vi "getOutputGain.vi"(8 "error in (no error)":errorcluster, 11 "Instrument.LockinAPI in":refnum<class "Instrument.LockinAPI.lvclass">) -> (0 "error out":errorcluster, 2 "OutputGain":dbl[](array[numeric]), 3 "Instrument.LockinAPI out":refnum<class "Instrument.LockinAPI.lvclass">)   [LabVIEW 2019, in "Instrument.LockinAPI.lvclass"]
doc: "API to get the AI waveforms.\n\nIf address=\"\", this API reads from localhost\nIf address is remote lockin, you need to add this computer to allowed whitelist on the lockin computer you are trying to access."
uses:
  Instrument.LockinAPI.lvclass
  C:/Users/patrick/Documents/GitHub/Instrument-Framework/lvsrc/Framework/Instrument/Instrument.lvclass
  Typedefs/LockinAPI.Commands--Enum.ctl
  00037c6a-def5-4a33-8a82-3535220e14b4.vi
  00037c6a-def5-4a33-8a82-3535220e14b4.vi/72857e9d-b6a5-4918-84de-0a0220085fa5.vi
  00037c6a-def5-4a33-8a82-3535220e14b4.vi/b18f0c14-d6dd-4c6b-8b21-3f3829313509.vi
  <vilib>/Utility/Data Type/Get Type Information.vi
  <vilib>/JDP Science/JSONtext/JSON text to Variant.vi
  <vilib>/JDP Science/JSONtext/LVClass Serializer/JSONtext LVClass Serializer.lvclass
  Instrument/Instrument.lvclass
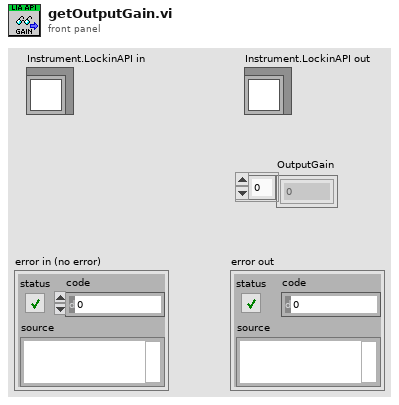
[diagram p1: front panel]
types:
  T1 = typedef "Instrument.LockinAPI.lvclass/LockinAPI.Commands--Enum.ctl" = enum16{"setAI", "setAO", "setAO_Amplitude", "setAO_DC", "setAO_Frequency", "setAO_Phase", "setAO_Function", "setAO_I+", "setREF", "setREF_Frequency", "setREF_Phase", "setREF_TC", "setREF_Roll-Off", "setDAQ", "setSampling", "setOffset", "setState", "getState", "getAO", "getAI", "getResults", "getSampling", "getAOconfig", "getREFconfig", "setInputGain", "setOutputGain", "getInputGain", "getOutputGain", "setSamplingMode", "getSamplingMode", "setSweep", "setSweepTime", "setSweepTable", "getStatus", "getSweepResults", "getSweepWaveforms", "startSweep", "stopSweep", "setAUX", "getAUX"}
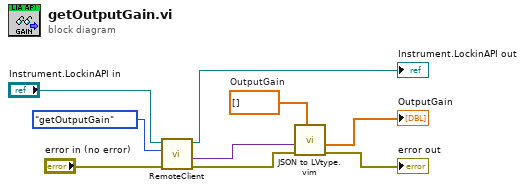
[diagram p0: block diagram]
diagram:
  w5 = dbl[] []  # OutputGain
  n1 = call "RemoteClient.vi"("error in (no error)"="error in (no error)", "Command in"=LockinAPI.Commands--Enum."getOutputGain" ("Command"), "Instrument in"="Instrument.LockinAPI in") -> ("error out"=w2:errorcluster, "Data out"=w4:variant, "Instrument out"=→"Instrument.LockinAPI out":refnum<class "Instrument.LockinAPI.lvclass">)  [unwired: 5 in, 1 out]
  n2 = call "JSON to LVtype.vim"("type"=w5, "error in (no error)"=w2, "JSON Data in"=w4) -> ("error out"=→"error out":errorcluster, "Data out"=→"OutputGain":dbl[])  [unwired: 7 in]
